vi "Collect.vi"(8 "error in (no error)":errorcluster, 11 "Process Collector in":refnum<class "Process Collector.lvclass">) -> (0 "error out":errorcluster, 2 "Metrics":refnum<data-value>[](array[refnum]), 3 "Process Collector out":refnum<class "Process Collector.lvclass">)   [LabVIEW 2020, in "Collector.lvlib" / "Process Collector.lvclass"]
uses:
  Process Collector.lvclass
  metrics/metric/Metric.lvclass
  metrics/gauge/Gauge.lvclass
  Process Collector.lvclass/Process Collector.ctl
  generic collector/Default Collector.lvclass
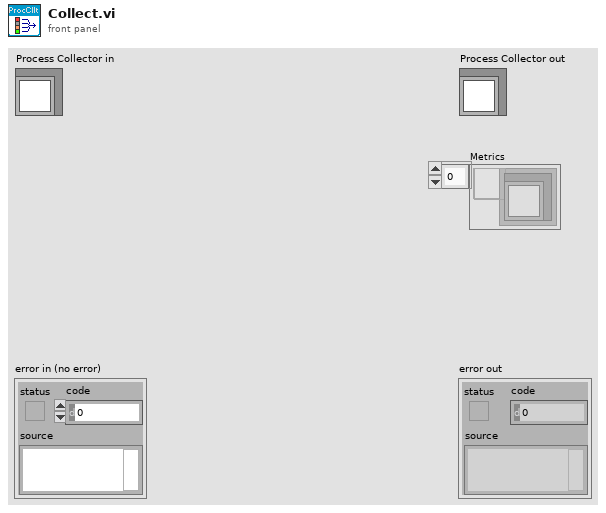
[diagram p1: front panel]
types:
  T1 = enum16{"seconds", "milliseconds", "microseconds"}
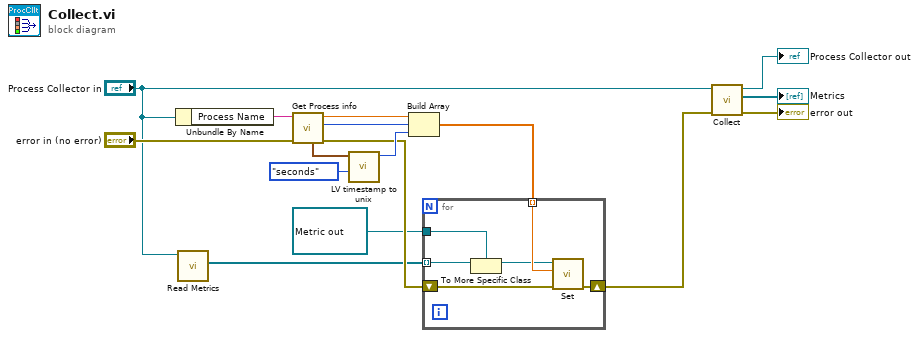
[diagram p0: block diagram]
diagram:
  n1 = Unbundle By Name("Process Collector in") -> ("Process Name"=w16:string)
  n2 = call-dynamic "Read Metrics.vi"("Default Collector in"="Process Collector in") -> ("Metrics"=w2:refnum<data-value>[])  [unwired: 8 in, 2 out]
  n3 = call "Get Process info.vi"("error in (no error)"="error in (no error)", "processName"=w16) -> ("error out"=w5:errorcluster, "VirtualMem Size"=w11:i64, "Total CPU Seconds"=w12:dbl, "StartTime"=w14:timestamp)  [unwired: 5 in, 1 out]
  n4 = call "LV timestamp to unix.vi"("Precision (ms)"=T1."seconds", "Timestamp"=w14) -> ("Unix epoch time"=w10:u64)  [unwired: 9 in]
  n5 = Build Array(w12, w11, w10) -> (w9:dbl[])
  n6 = for {
    tunnel: w9 -> [w22] mode=indexing
    shift-right: [w21] -> w3
    shift-left: w5 -> [w20]
    tunnel: w2 -> [w19] mode=indexing
    tunnel: refnum<data-value> refnum ("Gauge Ref") -> [w18]
    n7 = To More Specific Class(target class=w18, reference=w19) -> (specific class reference=w17:refnum<data-value>)  [unwired: 1 in, 1 out]
    n8 = call "Set.vi"("error in (no error)"=w20, "Value"=w22, "Gauge Ref"=w17) -> ("error out"=w21:errorcluster)  [unwired: 7 in, 1 out]
  }
  n9 = call-parent "Collect.vi"("error in (no error)"=w3, "Default Collector in"="Process Collector in") -> ("error out"=→"error out":errorcluster, "Metrics"=→"Metrics":refnum<data-value>[], "Default Collector out"=→"Process Collector out":refnum<class "Process Collector.lvclass">)  [unwired: 7 in]
